vi "_UtilsRandom2DU64Array.vi"(1 "random array size":i32=100, 2 "factor":dbl=1.0) -> (0 "random array":i64[][](array[numeric]))   [LabVIEW 2014, in "examples.lvlib"]
uses:
  examples.lvlib
  _UtilsRandomU64Array.vi
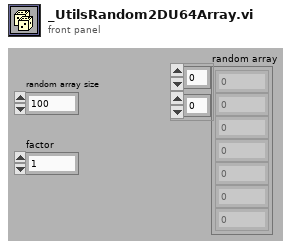
[diagram p1: front panel]
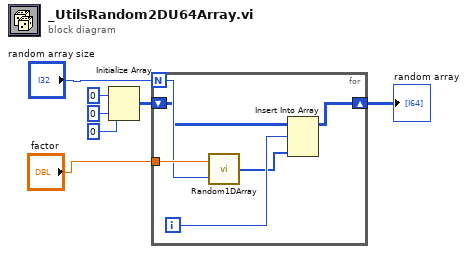
[diagram p0: block diagram]
diagram:
  n1 = Initialize Array(u64 0 ("element"), 0 ("dimension size"), 0 ("dimension size")) -> (w5:u64[][])
  n2 = for {
    N: "random array size" -> [w12]
    tunnel: "factor" -> [w13]
    shift-right: [w8] -> w4
    shift-left: w5 -> [w9]
    i -> [w11]
    n3 = call-poly "Random1DArray.vi"("array size"=w12, "factor"=w13) -> ("array"=w10:u64[])
    n4 = Insert Into Array(array=w9, index (row)=w11, new element=w10) -> (w8:u64[][])  [unwired: 1 in]
  }
  "random array" <- w4
